vi "GetState.vi"(8 "error in (no error)":errorcluster, 11 "reference in":refnum<class "Switch_MotorP5.lvclass">) -> (0 "error out":errorcluster, 1 "States":bool[](array[boolean]), 2 "Routes":string[](array[string]), 3 "reference in":refnum<class "Switch_MotorP5.lvclass">)   [LabVIEW 2022 SP3, in "Switch_MotorP5.lvlib" / "Switch_MotorP5.lvclass"]
uses:
  Switch_MotorP5.lvclass
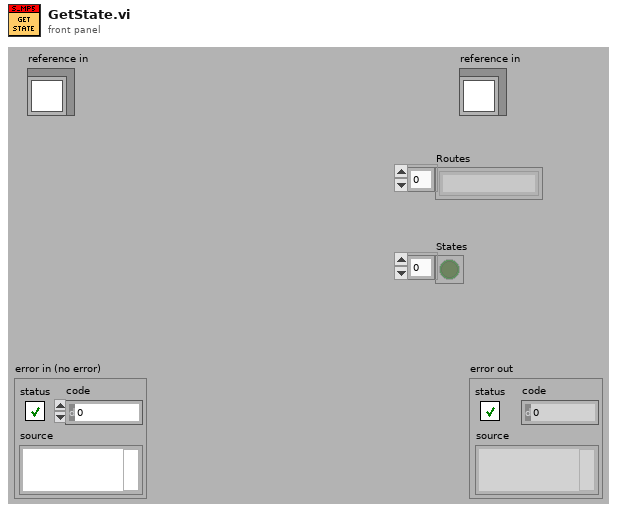
[diagram p1: front panel]
types:
  T1 = typedef "Switch_MotorP5.lvlib/Switch_MotorP5.lvclass/ObjectAttributes.ctl" = cluster{"Config":T2, "VISA":refnum<visa-resource-name>, "RPM":i32, "States":bool[], "UpdateEvent":refnum<user-event>, "Motor":enum32{"M1", "M2", "M3", "M4", "M5", "M6", "M7", "M8"}}
  T2 = typedef "Switch_MotorP5.lvlib/Switch_MotorP5.lvclass/Config.ctl" = cluster{"COM":refnum<visa-resource-name>, "SwitchMap":cluster{"Name":string, "Description":string, "Group":string, "IsGroup":bool, "Motor":enum32{"M1", "M2", "M3", "M4", "M5", "M6", "M7", "M8", "NA"}}[], "Sim":bool}
  T3 = cluster{"Name":string, "Description":string, "Group":string, "IsGroup":bool, "Motor":enum32{"M1", "M2", "M3", "M4", "M5", "M6", "M7", "M8", "NA"}}[]
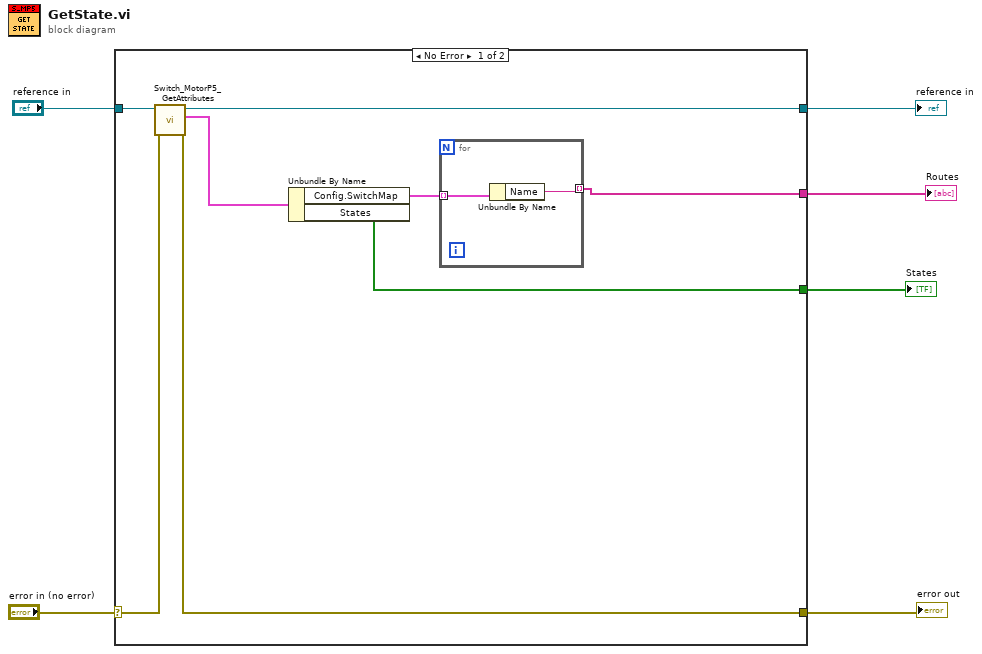
[diagram p0: block diagram]
diagram:
  n1 = case shown="No Error" "error in (no error)" {
    selector: "error in (no error)" -> [w14 w18]
    tunnel: [w12 w18] -> w5
    tunnel: [w10 w17] -> w3
    tunnel: "reference in" -> [w11 w17]
    tunnel: [w8 _] -> w2
    tunnel: [w7 _] -> w1
    frame No Error {
      n2 = call "Switch_MotorP5_GetAttributes.vi"("error in (no error)"=w14, "reference in"=w11) -> ("error out"=w12:errorcluster, "Data"=w13:T1, "reference out"=w10:refnum<class "Switch_MotorP5.lvclass">)  [unwired: 6 in, 1 out]
      n3 = Unbundle By Name(w13) -> ("Config.SwitchMap"=w9:T3, "States"=w7:bool[])
      n4 = for {
        tunnel: w9 -> [w16] mode=indexing
        tunnel: [w15] -> w8 mode=indexing
        n5 = Unbundle By Name(w16) -> ("Name"=w15:string)
      }
    }
    frame Error {
    }
  }
  "error out" <- w5
  "reference in" <- w3
  "Routes" <- w2
  "States" <- w1
